vi "Bind Timestamp.vi"(8 "error in (no error)":errorcluster, 10 "Time Stamp":timestamp, 11 "SQL Statement in":refnum<class "SQL Statement.lvclass">) -> (0 "error out":errorcluster, 3 "SQL Statement out":refnum<class "SQL Statement.lvclass">)   [LabVIEW 2013, in "SQLiteSupport.lvlib" / "SQL Statement.lvclass"]
doc: "Bind a LabVIEW Timestamp as a 128 bit BLOB."
uses:
  SQL Statement.lvclass
  SQL Statement.lvclass/SQL Statement.ctl
  Error Message.vi
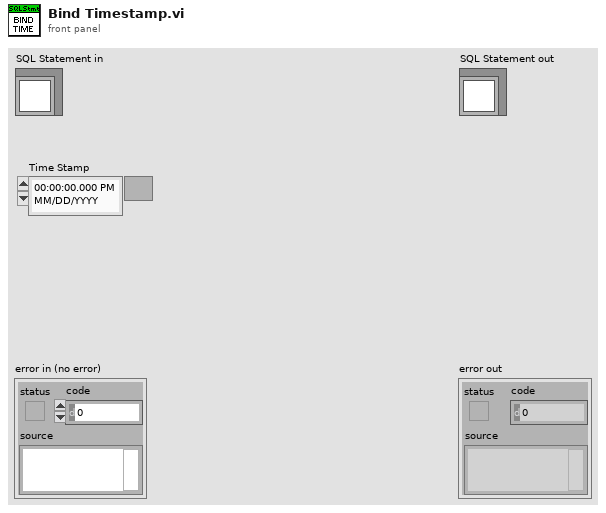
[diagram p1: front panel]
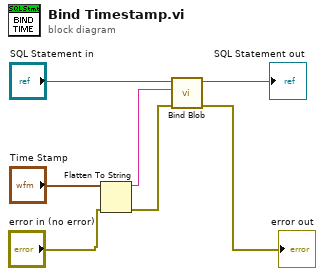
[diagram p0: block diagram]
diagram:
  n1 = Flatten To String(anything="Time Stamp", error in (no error)="error in (no error)") -> (data string=w3:string, error out=w1:errorcluster)  [unwired: 2 in, 1 out]
  n2 = call "Bind Blob.vi"("error in (no error)"=w1, "Blob"=w3, "SQL Statement in"="SQL Statement in") -> ("error out"=→"error out":errorcluster, "SQL Statement out"=→"SQL Statement out":refnum<class "SQL Statement.lvclass">)  [unwired: 7 in]
